vi "Zaber A Series XYZ List.vi"(8 "error constant":errorcluster, 9 "Read Coordinates from CSV":path, 11 "VISA resource name":refnum<visa-resource-name>) -> (0 "error out":errorcluster)   [LabVIEW 2018, in "Stage Actor.lvlib"]
doc: "This example moves a system of up to three axes through a list of co-ordinates. It uses the Move command as well as the Poll Until Idle library VI to co-ordinate the timing of the movements of the stages."
uses:
  Stage Actor.lvlib
  <vilib>/Utility/file.llb/Read Delimited Spreadsheet (string).vi
  <instrlib>/Zaber A Series/Zaber A Series.lvlib
panel:
  in  "Z-Axis Microstep Size (0)":dbl=0.047625
  in  "Z Device and Axis (03)":string="03"
  in  "Units (0: microsteps)":u16(ring)=2 items=["microsteps", "microns", "millimeters", "inches"]
  in  "Movement Type (0: relative)":u16(ring) items=["relative", "absolute"]
  in  "Y-Axis Microstep Size (0)":dbl=0.047625
  in  "XYZ Positions":string[][](table)
  in  "Y Device and Axis (02)":string="02"
  in  "X Device and Axis (01)":string="01"
  in  "X-Axis Microstep Size (0)":dbl=0.047625
  # "(c) 2017 Zaber Technologies.  ALL RIGHTS RESERVED."
  # "This example demonstrates how you can move between co-ordinates. Before running, enter all of the XYZ points you'd like your stages to move to and the VISA resource name of your conenction. Make sure the units of your positions match the units dropdown. Also ensure that the Axis numbers correspond to your device numbers. Finally enter the microstep sizes of the devices if you are using something other than microsteps.\n\nEnter a file path in the Read Coordinates from CSV field if you'd like to use a spreadsheet to load the points.\n\nThis example can be used for one or two axes only by omitting coordinates. Only non-empty fields will be read."
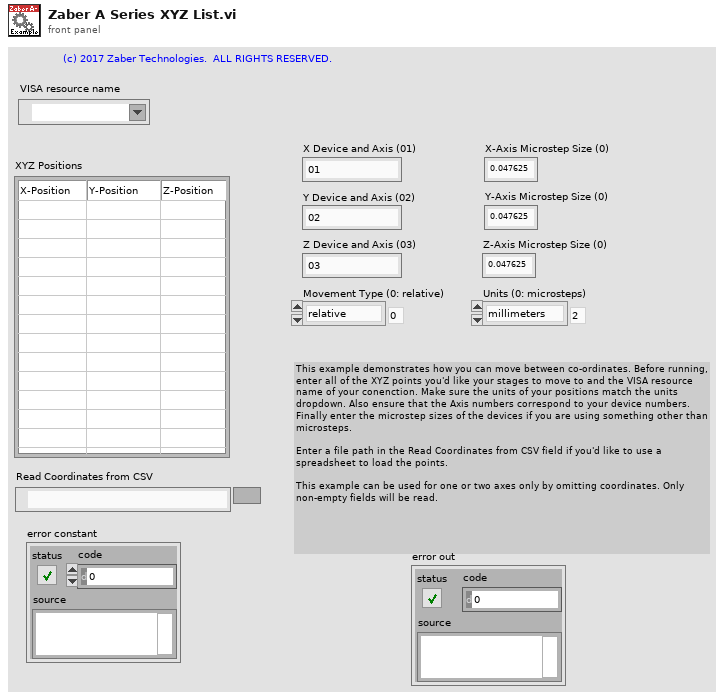
[diagram p1: front panel]
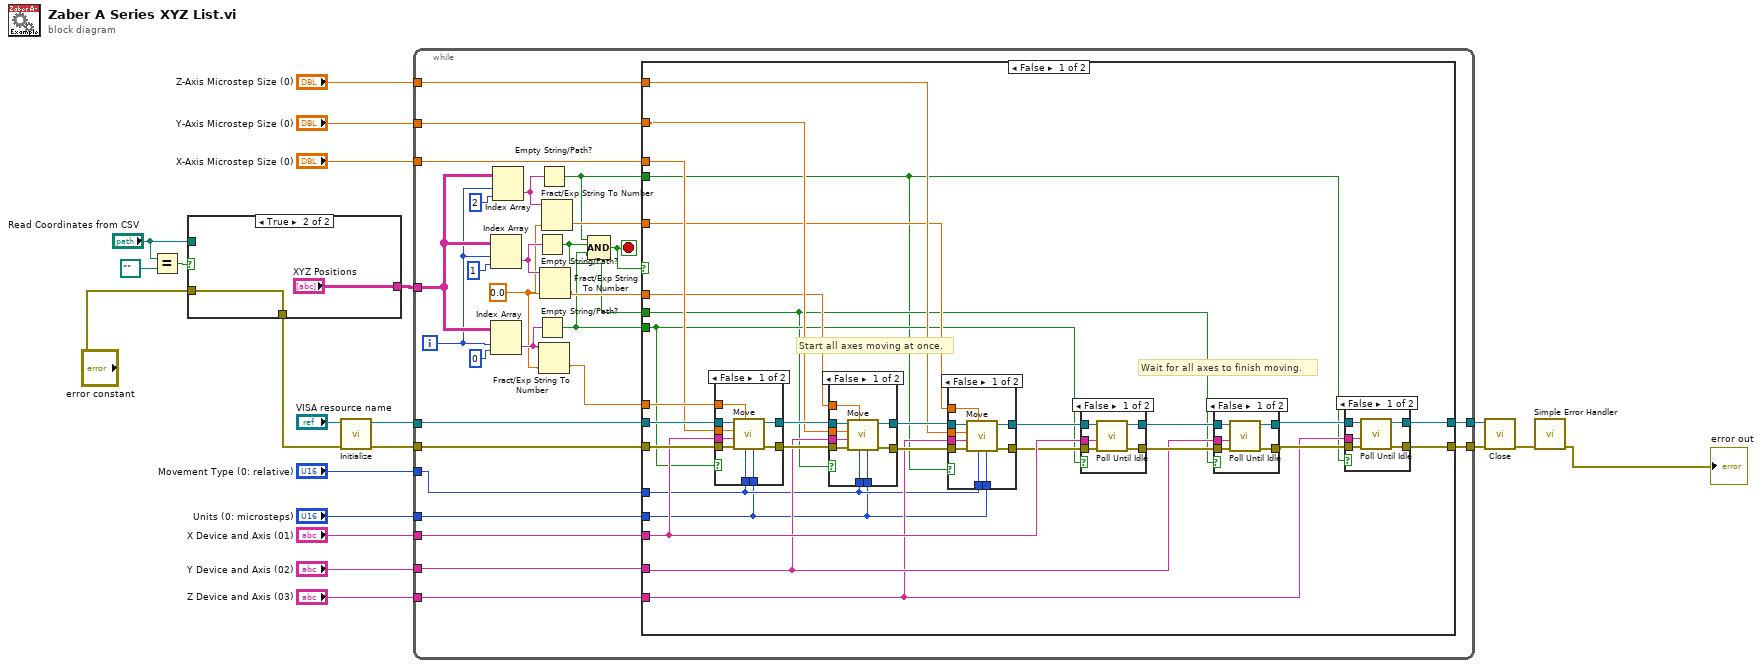
[diagram p0: block diagram]
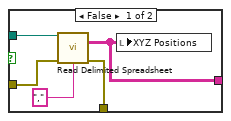
[diagram p2: hidden frame]
diagram:
  n1 = Equal?(x="Read Coordinates from CSV", y=path "") -> (x = y?=w4:bool)
  n2 = case shown="True" w4 {
    tunnel: "Read Coordinates from CSV" -> [w25 _]
    tunnel: [w24 "XYZ Positions"] -> w7
    tunnel: "error constant" -> [w23 w27]
    tunnel: [w22 w27] -> w2
    frame False {
      n3 = call-poly <vilib>:"Read Delimited Spreadsheet.vi"("file path (dialog if empty)"=w25, "error in (no error)"=w23, "delimiter (\\t)"="," ("delimiter (\\t)")) -> ("all rows"=w24:string[][], "error out"=w22:errorcluster)  [unwired: 7 in, 4 out]
      n4 = local write "XYZ Positions"(w24) -> ()
    }
    frame True {
    }
  }
  n5 = call <instrlib>:"Initialize.vi"("error in (no error)"=w2, "VISA resource name"="VISA resource name") -> ("error out"=w15:errorcluster, "VISA resource name out"=w20:refnum<visa-resource-name>)  [unwired: 8 in]
  n6 = while {
    tunnel: w20 -> [w56]
    tunnel: w7 -> [w37]
    tunnel: "Units (0: microsteps)" -> [w53]
    tunnel: "Movement Type (0: relative)" -> [w52]
    tunnel: "Y Device and Axis (02)" -> [w51]
    tunnel: "X Device and Axis (01)" -> [w50]
    tunnel: w15 -> [w49]
    tunnel: [w48] -> w14
    tunnel: [w47] -> w13
    tunnel: "Y-Axis Microstep Size (0)" -> [w46]
    tunnel: "X-Axis Microstep Size (0)" -> [w45]
    tunnel: "Z Device and Axis (03)" -> [w40]
    tunnel: "Z-Axis Microstep Size (0)" -> [w39]
    i -> [w36]
    stop <- w32 stop-if-true
    w35 = 0.0
    n7 = Index Array(array=w37, index (row)=w36, index (col)=1 ("disabled index (col)")) -> (element=w44:string)
    n8 = Index Array(array=w37, index (row)=w36, index (col)=0 ("disabled index (col)")) -> (element=w41:string)
    n9 = Index Array(array=w37, index (row)=w36, index (col)=2 ("disabled index (col)")) -> (element=w33:string)
    n10 = Empty String/Path?(string/path=w44) -> (empty?=w29:bool)
    n11 = Empty String/Path?(string/path=w41) -> (empty?=w30:bool)
    n12 = Empty String/Path?(string/path=w33) -> (empty?=w31:bool)
    n13 = Fract/Exp String To Number(string=w41, default (0 dbl)=w35) -> (number=w42:dbl)  [unwired: 2 in, 1 out]
    n14 = Fract/Exp String To Number(string=w44, default (0 dbl)=w35) -> (number=w43:dbl)  [unwired: 2 in, 1 out]
    n15 = Fract/Exp String To Number(string=w33, default (0 dbl)=w35) -> (number=w34:dbl)  [unwired: 2 in, 1 out]
    n16 = Compound Arithmetic op=AND(w31, w29, w30) -> (w32:bool)
    n17 = case shown="False" w32 {
      tunnel: w53 -> [w64 _]
      tunnel: w56 -> [w83 w139]
      tunnel: w50 -> [w74 _]
      tunnel: w51 -> [w67 _]
      tunnel: w52 -> [w65 _]
      tunnel: w42 -> [w84 _]
      tunnel: w43 -> [w61 _]
      tunnel: w49 -> [w82 w140]
      tunnel: [w79 w140] -> w47
      tunnel: [w80 w139] -> w48
      tunnel: w46 -> [w63 _]
      tunnel: w45 -> [w81 _]
      tunnel: w40 -> [w66 _]
      tunnel: w39 -> [w62 _]
      tunnel: w34 -> [w60 _]
      tunnel: w31 -> [w57 _]
      tunnel: w30 -> [w59 _]
      tunnel: w29 -> [w58 _]
      frame False {
        # "Start all axes moving at once."
        # "Wait for all axes to finish moving."
        n18 = case shown="False" w59 {
          tunnel: w64 -> [w115 _]
          tunnel: [w114 w117] -> w73
          tunnel: w65 -> [w113 _]
          tunnel: w84 -> [w112 _]
          tunnel: w83 -> [w111 w117]
          tunnel: w82 -> [w110 w116]
          tunnel: [w109 w116] -> w72
          tunnel: w81 -> [w108 _]
          tunnel: w74 -> [w107 _]
          frame False {
            n19 = call <instrlib>:"Move.vi"("Units (0: microsteps)"=w115, "Movement Type (0: relative)"=w113, "Move Distance (0)"=w112, "error in (no error)"=w110, "Device and Axis"=w107, "Microstep Size (0)"=w108, "VISA resource name"=w111) -> ("error out"=w109:errorcluster, "VISA resource name out"=w114:refnum<visa-resource-name>)  [unwired: 3 in]
          }
          frame True {
          }
        }
        n20 = case shown="False" w58 {
          tunnel: w64 -> [w104 _]
          tunnel: [w103 w106] -> w71
          tunnel: w65 -> [w102 _]
          tunnel: w61 -> [w101 _]
          tunnel: w73 -> [w100 w106]
          tunnel: w72 -> [w97 w105]
          tunnel: [w96 w105] -> w70
          tunnel: w63 -> [w99 _]
          tunnel: w67 -> [w98 _]
          frame False {
            n21 = call <instrlib>:"Move.vi"("Units (0: microsteps)"=w104, "Movement Type (0: relative)"=w102, "Move Distance (0)"=w101, "error in (no error)"=w97, "Device and Axis"=w98, "Microstep Size (0)"=w99, "VISA resource name"=w100) -> ("error out"=w96:errorcluster, "VISA resource name out"=w103:refnum<visa-resource-name>)  [unwired: 3 in]
          }
          frame True {
          }
        }
        n22 = case shown="False" w57 {
          tunnel: w64 -> [w93 _]
          tunnel: [w92 w95] -> w69
          tunnel: w65 -> [w91 _]
          tunnel: w60 -> [w90 _]
          tunnel: w71 -> [w89 w95]
          tunnel: w70 -> [w88 w94]
          tunnel: [w87 w94] -> w68
          tunnel: w62 -> [w86 _]
          tunnel: w66 -> [w85 _]
          frame False {
            n23 = call <instrlib>:"Move.vi"("Units (0: microsteps)"=w93, "Movement Type (0: relative)"=w91, "Move Distance (0)"=w90, "error in (no error)"=w88, "Device and Axis"=w85, "Microstep Size (0)"=w86, "VISA resource name"=w89) -> ("error out"=w87:errorcluster, "VISA resource name out"=w92:refnum<visa-resource-name>)  [unwired: 3 in]
          }
          frame True {
          }
        }
        n24 = case shown="False" w59 {
          tunnel: w69 -> [w136 w138]
          tunnel: w74 -> [w135 _]
          tunnel: w68 -> [w134 w137]
          tunnel: [w133 w137] -> w75
          tunnel: [w132 w138] -> w76
          frame False {
            n25 = call <instrlib>:"Poll Until Idle.vi"("error in (no error)"=w134, "Device and Axis"=w135, "VISA resource name"=w136) -> ("error out"=w133:errorcluster, "VISA resource name out"=w132:refnum<visa-resource-name>)  [unwired: 7 in]
          }
          frame True {
          }
        }
        n26 = case shown="False" w58 {
          tunnel: w76 -> [w129 w131]
          tunnel: w67 -> [w128 _]
          tunnel: w75 -> [w127 w130]
          tunnel: [w126 w130] -> w77
          tunnel: [w125 w131] -> w78
          frame False {
            n27 = call <instrlib>:"Poll Until Idle.vi"("error in (no error)"=w127, "Device and Axis"=w128, "VISA resource name"=w129) -> ("error out"=w126:errorcluster, "VISA resource name out"=w125:refnum<visa-resource-name>)  [unwired: 7 in]
          }
          frame True {
          }
        }
        n28 = case shown="False" w57 {
          tunnel: w78 -> [w122 w124]
          tunnel: w66 -> [w121 _]
          tunnel: w77 -> [w120 w123]
          tunnel: [w119 w123] -> w79
          tunnel: [w118 w124] -> w80
          frame False {
            n29 = call <instrlib>:"Poll Until Idle.vi"("error in (no error)"=w120, "Device and Axis"=w121, "VISA resource name"=w122) -> ("error out"=w119:errorcluster, "VISA resource name out"=w118:refnum<visa-resource-name>)  [unwired: 7 in]
          }
          frame True {
          }
        }
      }
      frame True {
      }
    }
  }
  n30 = call <instrlib>:"Close.vi"("error in (no error)"=w13, "VISA resource name"=w14) -> ("error out"=w12:errorcluster)  [unwired: 9 in]
  n31 = call <vilib>:"Simple Error Handler.vi"("error in (no error)"=w12) -> ("error out"=→"error out":errorcluster)  [unwired: 4 in, 4 out]
